vi "Read.vi"(6 "Read Length":u32, 8 "Error In":errorcluster, 9 "Offset":u32 format="%.0x", 10 "Index Group":u32 format="%.0x", 11 "AMS Connection In":T2) -> (0 "Error Out":errorcluster, 2 "ADS Error":T1 items=["NoError"=0, "InternalError"=1, "NoRTime"=2, "LockedMemoryError"=3, "MailBoxError"=4, "WrongHMsg"=5, "TargetPortNotFound"=6, "TargetMachineNotFound"=7, "UnknownCommandID"=8, "BadTaskID"=9, "NoIO"=10, "UnknownAmsCommand"=11, "Win32Error"=12, "PortNotConnected"=13, "InvalidAmsLength"=14, "InvalidAmsNetID"=15, "AmsSyncAmsError"=22, "AmsSyncNoIndexMap"=23, "InvalidAmsPort"=24, "NoMemory"=25, "TCPSendError"=26, "HostUnreachable"=27, "NoLockedMemory"=1280, "MailboxFull"=1282, "DeviceError"=1792, "DeviceServiceNotSupported"=1793, "DeviceInvalidGroup"=1794, "DeviceInvalidOffset"=1795, "DeviceInvalidAccess"=1796, "DeviceInvalidSize"=1797, "DeviceInvalidData"=1798, "DeviceNotReady"=1799, "DeviceBusy"=1800, "DeviceInvalidContext"=1801, "DeviceNoMemory"=1802, "DeviceInvalidParam"=1803, "DeviceNotFound"=1804, "DeviceSyntaxError"=1805, "DeviceIncompatible"=1806, "DeviceExists"=1807, "DeviceSymbolNotFound"=1808, "DeviceSymbolVersionInvalid"=1809, "DeviceInvalidState"=1810, "DeviceTransModeNotSupported"=1811, "DeviceNotifyHandleInvalid"=1812, "DeviceClientUnknown"=1813, "DeviceNoMoreHandles"=1814, "DeviceInvalidWatchsize"=1815, "DeviceNotInitialized"=1816, "DeviceTimeOut"=1817, "DeviceNoInterface"=1818, "DeviceInvalidInterface"=1819, "DeviceInvalidCLSID"=1820, "DeviceInvalidObjectID"=1821, "ClientError"=1856, "ClientInvalidParameter"=1857, "ClientListEmpty"=1858, "ClientVariableInUse"=1859, "ClientDuplicateInvokeID"=1860, "ClientSyncTimeOut"=1861, "ClientW32OR"=1862, "ClientTimeoutInvalid"=1863, "ClientPortNotOpen"=1864, "ClientNoAmsAddr"=1865, "ClientSyncInternal"=1872, "ClientAddHash"=1873, "ClientRemoveHash"=1874, "ClientNoMoreSymbols"=1875, "ClientSyncResInvalid"=1876, "ClientSyncPortLocked"=1877, "ClientQueueFull"=1878], 3 "Data":u8[](array[numeric]))   [LabVIEW 2017, in "TwinCAT ADS.lvlib"]
uses:
  TwinCAT ADS.lvlib
  Low Level/TypeDefs/AMS Connection.ctl
  Low Level/TypeDefs/AMS.ctl
  Low Level/TypeDefs/ADS Error.ctl
  Low Level/TypeDefs/Command Id.ctl
  Low Level/TypeDefs/State Flag.ctl
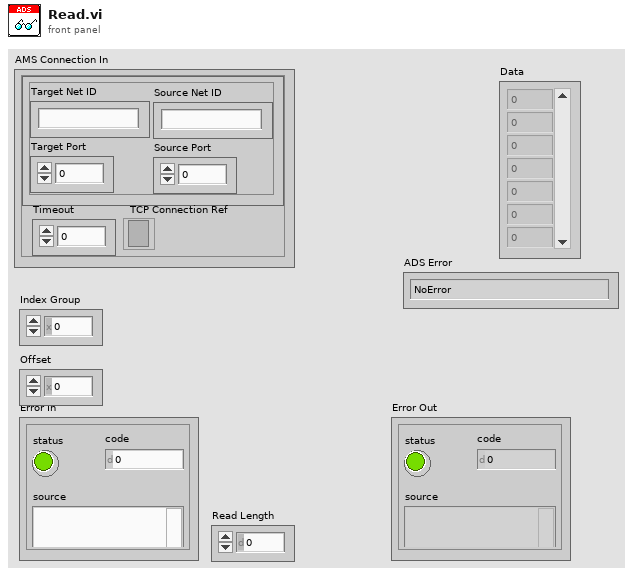
[diagram p1: front panel]
types:
  T1 = typedef "TwinCAT ADS.lvlib/ADS Error.ctl" = i32
  T2 = typedef "TwinCAT ADS.lvlib/AMS Connection.ctl" = cluster{"AMS":T3, "Timeout":i32, "TCP Connection Ref":refnum<k5>}
  T3 = typedef "TwinCAT ADS.lvlib/AMS.ctl" = cluster{"Target Net ID":string, "Target Port":u16, "Source Net ID":string, "Source Port":u16}
  T4 = enum16{"Standard", "Buffered", "CRLF", "Immediate"}
  T5 = typedef "TwinCAT ADS.lvlib/State Flag.ctl" = u16
  T6 = typedef "TwinCAT ADS.lvlib/Command Id.ctl" = enum16{"Invalid", "ADS Read Device Info", "ADS Read", "ADS Write", "ADS Read State", "ADS Write Control", "ADS Add Device Notification", "ADS Delete Device Notification", "ADS Device Notification", "ADS Read Write"}
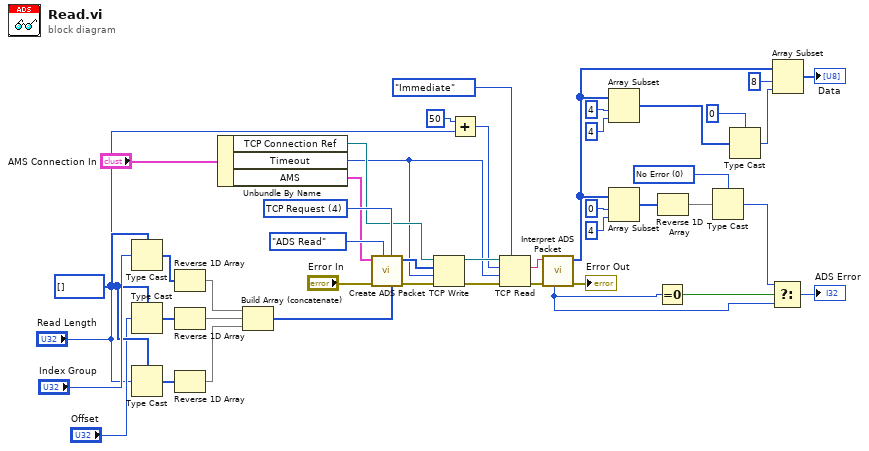
[diagram p0: block diagram]
diagram:
  w23 = T1 0 items=["No Error"] ("Enum")
  w32 = u8[] [] ("bytes to read")
  w44 = T5 4 items=["TCP Request"=4, "TCP Response"=5, "UDP Request"=68, "UDP Respone"=69] ("State Flag")
  n1 = Type Cast(type=w32, x="Index Group") -> (*(type *) &x=w30:u8[])
  n2 = Type Cast(type=w32, x="Offset") -> (*(type *) &x=w29:u8[])
  n3 = Type Cast(type=w32, x="Read Length") -> (*(type *) &x=w28:u8[])
  n4 = Reverse 1D Array(array=w30) -> (reversed array=w13:u8[])
  n5 = Reverse 1D Array(array=w29) -> (reversed array=w12:u8[])
  n6 = Reverse 1D Array(array=w28) -> (reversed array=w11:u8[])
  n7 = Unbundle By Name("AMS Connection In") -> ("TCP Connection Ref"=w3:refnum<k5>, "Timeout"=w2:i32, "AMS"=w4:T3)
  n8 = Build Array (concatenate)(w13, w12, w11) -> (w27:u8[])
  n9 = call "Create ADS Packet.vi"("Data"=w27, "State Flag"=w44, "Command ID"=Command_Id."ADS Read", "Error In"="Error In", "AMS"=w4) -> ("Error Out"=w41:errorcluster, "ADS Packet"=w43:u8[])  [unwired: 5 in]
  n10 = TCP Write(connection ID=w3, data in=w43, error in (no error)=w41, 9:w2) -> (connection ID out=w42:refnum<k5>, error out=w40:errorcluster)  [unwired: 1 out]
  n11 = Add(x=u32 50 ("bytes to read"), y="Read Length") -> (x+y=w15:u32)
  n12 = TCP Read(connection ID=w42, bytes to read=w15, error in (no error)=w40, 7:T4."Immediate" ("mode (standard)"), 9:w2) -> (data out=w35:string, error out=w36:errorcluster)  [unwired: 1 out]
  n13 = call "Interpret ADS Packet.vi"("Error In"=w36, "ADS Packet"=w35) -> ("Error Out"=→"Error Out":errorcluster, "Data"=w18:u8[], "ADS Error"=w6:T1)  [unwired: 3 in, 4 out]
  n14 = Array Subset(array=w18, index=4, length=4) -> (w20:u8[])
  n15 = Array Subset(array=w18, index=0, length=4) -> (w24:u8[])
  n16 = Equal To 0?(x=w6) -> (x = 0?=w8:bool)
  n17 = Reverse 1D Array(array=w24) -> (reversed array=w9:u8[])
  n18 = Type Cast(type=w23, x=w9) -> (*(type *) &x=w7:T1)
  n19 = Type Cast(type=u32 0 ("bytes to read"), x=w20) -> (*(type *) &x=w10:u32)
  n20 = Select(t=w7, s=w8, f=w6) -> (s? t:f=→"ADS Error":T1)
  n21 = Array Subset(array=w18, index=8, length=w10) -> (→"Data":u8[])
